vi "validate configuration.vi"(8 "error in":errorcluster, 11 "tag bus configurable plugin module configuration in":refnum<class "fixed channel tag bus module configuration.lvclass">) -> (0 "error out":errorcluster, 3 "tag bus configurable plugin module configuration out":refnum<class "fixed channel tag bus module configuration.lvclass">)   [LabVIEW 2013, in "fixed channel tag bus module configuration.lvclass"]
doc: "This function performs validation of the configuration. This function should be safe to call at any point and should not rely on anything in the runtime environment."
uses:
  fixed channel tag bus module configuration.lvclass
  <vilib>/NI/Tag Bus Module Framework/module configuration/TBM module configuration.lvclass
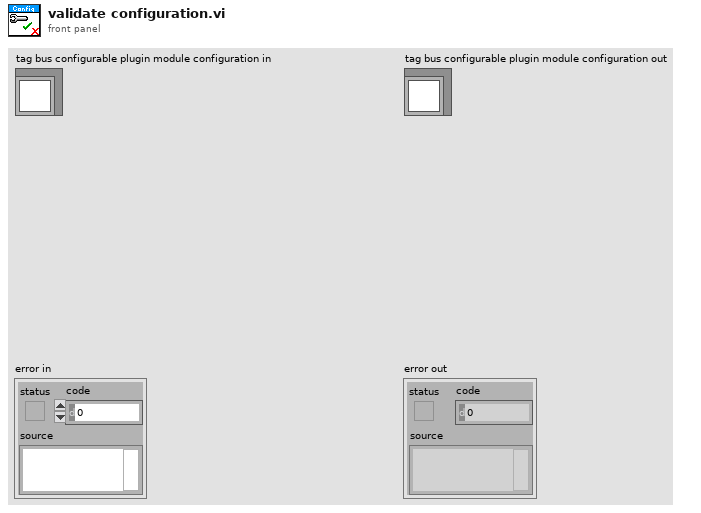
[diagram p1: front panel]
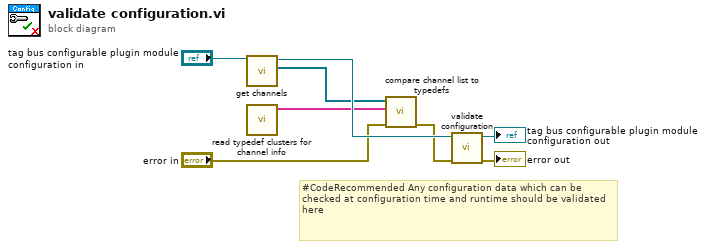
[diagram p0: block diagram]
diagram:
  # "#CodeRecommended Any configuration data which can be checked at configuration time and runtime should be validated here"
  n1 = call-dynamic "get channels.vi"("user tag bus module configuration In"="tag bus configurable plugin module configuration in") -> ("channels"=w4:refnum<class "TBM channel.lvclass">[], "user tag bus module configuration Out"=w5:refnum<class "fixed channel tag bus module configuration.lvclass">)  [unwired: 9 in]
  n2 = call "read typedef clusters for channel info.vi"() -> ("> Uncategorized name list >"=w3:string[])  [unwired: 9 in, 2 out]
  n3 = call "compare channel list to typedefs.vi"("error in"="error in", "> Uncategorized name list >"=w3, "configured channels in"=w4) -> ("error out"=w2:errorcluster)  [unwired: 7 in, 1 out]
  n4 = call-parent "validate configuration.vi"("error in"=w2, "configuration in"=w5) -> ("error out"=→"error out":errorcluster, "configuration out"=→"tag bus configurable plugin module configuration out":refnum<class "fixed channel tag bus module configuration.lvclass">)  [unwired: 8 in]
